vi "AM_Write_Volt.vi"(0 "VISA resource name":refnum<visa-resource-name>, 1 "Volt / V":dbl min=0.0 max=3.3, 2 "Delay / ms":u32, 3 "Enum":enum16{"Ch. A", "Ch. B"}(ring), 4 "error in (no error)":errorcluster) -> (5 "VISA resource name 2":refnum<visa-resource-name>, 6 "Cmd":string, 7 "error out":errorcluster)   [LabVIEW 2019]
doc: "Send a command to the Arduino Micro telling it to output a voltage between 0 and 5 V on channel A or channel B\n\nR. Sheehan 13 - 11 - 2020"
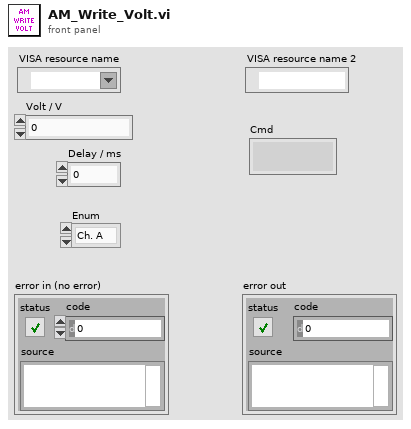
[diagram p1: front panel]
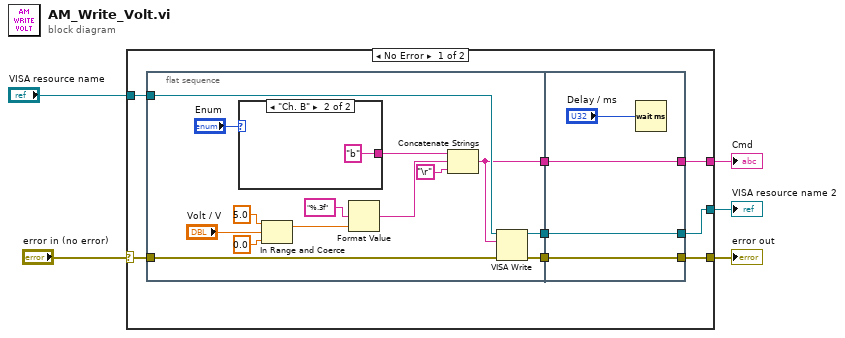
[diagram p0: block diagram]
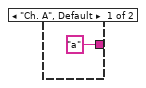
[diagram p2: hidden frame]
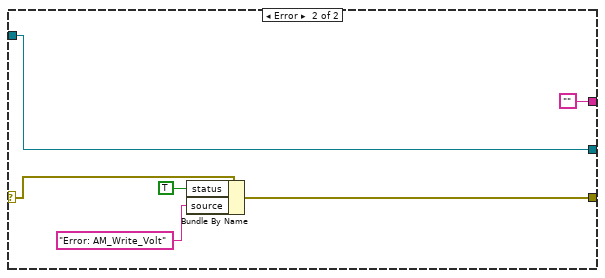
[diagram p3: hidden frame]
diagram:
  n1 = case shown="No Error" "error in (no error)" {
    selector: "error in (no error)" -> [w12 w39]
    tunnel: [w9 w38] -> w4
    tunnel: "VISA resource name" -> [w13 w35]
    tunnel: [w10 w35] -> w2
    tunnel: [w11 ""] -> w1
    frame No Error {
      n2 = flat-sequence {
        tunnel: w13 -> [w24]
        tunnel: w12 -> [w23]
        tunnel: [w22] -> w8
        tunnel: [w21] -> w7
        tunnel: [w20] -> w6
        tunnel: [w31] -> w9
        tunnel: [w32] -> w10
        tunnel: [w33] -> w11
        tunnel: w8 -> [w33]
        tunnel: w7 -> [w32]
        tunnel: w6 -> [w31]
        frame #0 {
          n3 = case shown="\"Ch. B\"" "Enum" {
            tunnel: ["a" ("string") "b" ("string")] -> w14
            frame "Ch. A", Default {
            }
            frame "Ch. B" {
            }
          }
          n4 = In Range and Coerce(upper limit=5.0, x="Volt / V", lower limit=0.0) -> (coerced(x)=w16:dbl)  [unwired: 1 out]
          n5 = Format Value(format string="%.3f", value (0)=w16) -> (output string=w25:string)  [unwired: 1 in]
          n6 = Concatenate Strings(w14, w25, "\r") -> (w22:string)
          n7 = VISA Write(VISA resource name=w24, write buffer=w22, error in (no error)=w23) -> (VISA resource name out=w21:refnum<visa-resource-name>, error out=w20:errorcluster)  [unwired: 1 out]
        }
        frame #1 {
          n8 = Wait (ms)(milliseconds to wait="Delay / ms") -> ()  [unwired: 1 out]
        }
      }
    }
    frame Error {
      n9 = Bundle By Name(cluster=w39, "status"=TRUE, "source"="Error: AM_Write_Volt") -> (w38:errorcluster)
    }
  }
  "error out" <- w4
  "VISA resource name 2" <- w2
  "Cmd" <- w1
